vi "from string array.vi"(8 "error in (no error)":errorcluster, 9 "String Array":string[][](array[string]), 10 "version":string, 11 "module configuration in":refnum<class "J1939 configuration.lvclass">) -> (0 "error out":errorcluster, 3 "module configuration out":refnum<class "J1939 configuration.lvclass">)   [LabVIEW 2017, in "J1939 configuration.lvclass"]
uses:
  J1939 configuration.lvclass
  Line.ctl
  <vilib>/NI/Tag Bus Module Framework/channel/TBM channel.lvclass
  <vilib>/NI/Tag Bus/tag/Data Type.ctl
  <vilib>/NI/Tag Bus Module Framework/channel/channel classification.ctl
  J1939 configuration.lvclass/J1939 configuration.ctl
  Write Lines.vi
  <vilib>/NI/Tag Bus/tag/tag descriptor.lvclass
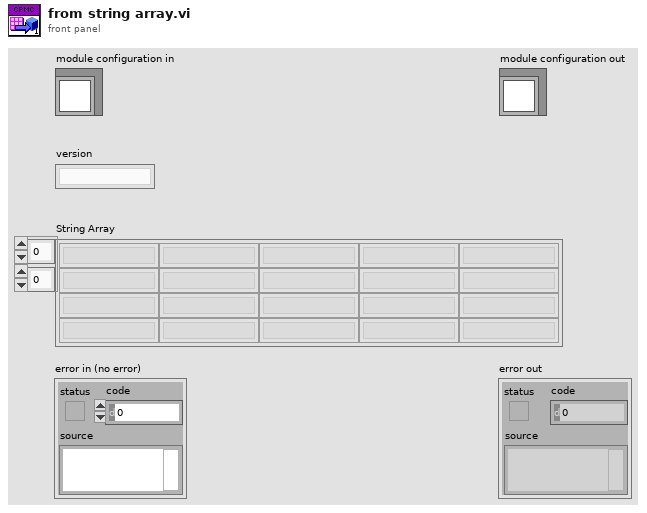
[diagram p1: front panel]
types:
  T1 = typedef "TBM channel.lvclass/channel classification.ctl" = enum16{"input data", "output data", "processing parameter", "processing result"}
  T2 = typedef "tag bus.lvlib/tag descriptor.lvclass/Data Type.ctl" = enum16{"Double", "Single", "I64", "I32", "I16", "I8", "U64", "U32", "U16", "U8", "Boolean", "String", "Array of Double", "Array of Single", "Array of I64", "Array of I32", "Array of I16", "Array of I8", "Array of U64", "Array of U32", "Array of U16", "Array of U8", "Array of Boolean", "Array of String"}
  T3 = typedef "J1939 configuration.lvclass/Line.ctl" = cluster{"channel":refnum<class "TBM channel.lvclass">, "XNET Signal":refnum<k21>}
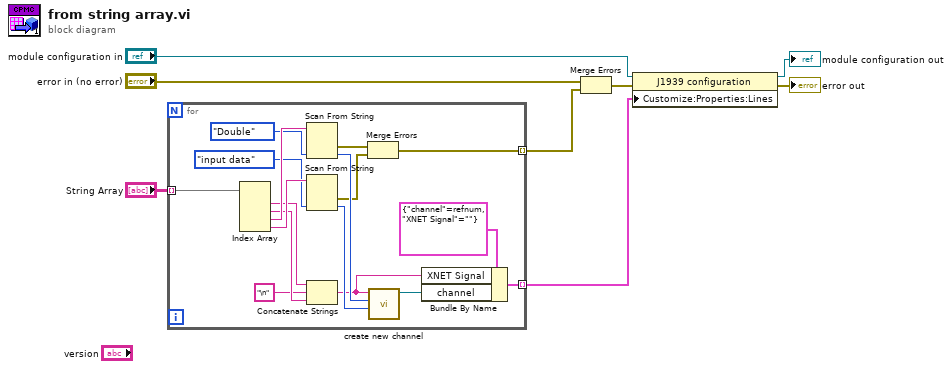
[diagram p0: block diagram]
diagram:
  n1 = for {
    tunnel: "String Array" -> [w23] mode=indexing
    tunnel: [w25] -> w5 mode=indexing
    tunnel: [w9] -> w2 mode=indexing
    n2 = Index Array(array=w23) -> (element #1=w14:string, element #2=w15:string, element #3=w22:string, element #4=w19:string)  [unwired: 4 in]
    n3 = Scan From String(input string=w22, default 1=Data_Type."Double" ("data type")) -> (error out=w11:errorcluster, output 1=w20:T2)  [unwired: 3 in, 2 out]
    n4 = Scan From String(input string=w19, default 1=channel_classification."input data" ("channel classification")) -> (error out=w10:errorcluster, output 1=w17:T1)  [unwired: 3 in, 2 out]
    n5 = Concatenate Strings(w14, "\n" ("search string/char (-)"), w15) -> (w13:string)
    n6 = Merge Errors(w11, w10) -> (w9:errorcluster)
    n7 = call <vilib>:"create new channel.vi"("channel classification"=w17, "data type"=w20, "channel name"=w13) -> ("channel"=w16:refnum<class "TBM channel.lvclass">)  [unwired: 8 in]
    n8 = Bundle By Name(cluster=T3 {"channel"=refnum, "XNET Signal"=""} ("Line"), "XNET Signal"=w13, "channel"=w16) -> (w25:T3)
  }
  n9 = Merge Errors("error in (no error)", w2) -> (w1:errorcluster)
  n10 = property class="J1939 configuration"(reference="module configuration in", error in=w1, "Customize:Properties:Lines"=w5) -> (reference out=→"module configuration out":refnum<class "J1939 configuration.lvclass">, error out=→"error out":errorcluster)
